vi "Compare Observable Values.vi"(1 "Value 2":string, 2 "Value 1":string, 3 "Comparison":string) -> (0 "Boolean":bool)   [LabVIEW 2020, in "CIRCUS_uServices.lvlib" / "Analysis Framework.lvclass"]
uses:
  Analysis Framework.lvclass
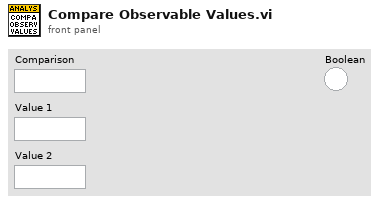
[diagram p1: front panel]
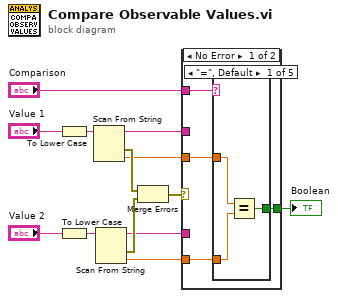
[diagram p0: block diagram]
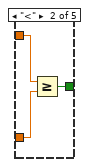
[diagram p2: hidden frame]
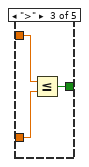
[diagram p3: hidden frame]
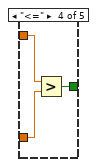
[diagram p4: hidden frame]
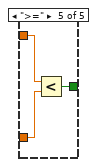
[diagram p5: hidden frame]
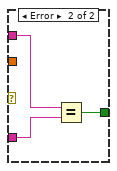
[diagram p6: hidden frame]
diagram:
  n1 = To Lower Case(string="Value 1") -> (all lower case string=w10:string)
  n2 = To Lower Case(string="Value 2") -> (all lower case string=w11:string)
  n3 = Scan From String(input string=w10) -> (remaining string=w2:string, error out=w9:errorcluster, output 1=w5:dbl)  [unwired: 4 in, 1 out]
  n4 = Scan From String(input string=w11) -> (remaining string=w1:string, error out=w8:errorcluster, output 1=w4:dbl)  [unwired: 4 in, 1 out]
  n5 = Merge Errors(w9, w8) -> (w3:errorcluster)
  n6 = case shown="No Error" w3 {
    tunnel: w4 -> [w16 _]
    tunnel: w5 -> [w17 _]
    tunnel: [w15 w35] -> w12
    tunnel: "Comparison" -> [w14 _]
    tunnel: w2 -> [_ w34]
    tunnel: w1 -> [_ w33]
    frame No Error {
      n7 = case shown="\"=\", Default" w14 {
        tunnel: w17 -> [w19 w23 w26 w29 w31]
        tunnel: w16 -> [w20 w22 w25 w28 w30]
        tunnel: [w18 w21 w24 w27 w32] -> w15
        frame "=", Default {
          n8 = Equal?(x=w19, y=w20) -> (x = y?=w18:bool)
        }
        frame "<" {
          n9 = Greater Or Equal?(x=w23, y=w22) -> (x >= y?=w21:bool)
        }
        frame ">" {
          n10 = Less Or Equal?(x=w26, y=w25) -> (x <= y?=w24:bool)
        }
        frame "<=" {
          n11 = Greater?(x=w29, y=w28) -> (0:w27:bool)
        }
        frame ">=" {
          n12 = Less?(x=w31, y=w30) -> (x < y?=w32:bool)
        }
      }
    }
    frame Error {
      n13 = Equal?(x=w34, y=w33) -> (x = y?=w35:bool)
    }
  }
  "Boolean" <- w12
